vi "Begin.vi"(8 "error in":errorcluster) -> (0 "error out":errorcluster)   [LabVIEW 2018]
doc: "Called before other user functions, this VI is expected to open initial I/O refnums, load in file data, and do all program initialization. Notice that the <B>error out</B> terminal is simply used for data flow. Wiring it to other structures or subVIs ensures that this VI runs first."
uses:
  <vilib>/Rock Robotics/WPI/DriverStation/WPI_DriverStationRobotMode2.ctl
  <vilib>/Rock Robotics/WPI/Joystick/WPI_JoystickDeviceEnum.ctl
  <vilib>/Rock Robotics/WPI/Solenoid/WPI_SolenoidChannel.ctl
  <vilib>/Rock Robotics/SystemInterfaces/DIO/FPGA_DIOChannel.ctl
  <vilib>/Rock Robotics/SystemInterfaces/DIO/FPGA_DIOPWMChannel.ctl
  Robot Global Data.vi
  <vilib>/Rock Robotics/WPI/Solenoid/WPI_SolenoidOpenSingle.vi
  <vilib>/Rock Robotics/WPI/Switch/WPI_SwitchOpenLimit.vi
  <vilib>/Rock Robotics/WPI/Utilities/WPI_GetSetVariantRefNum.vi
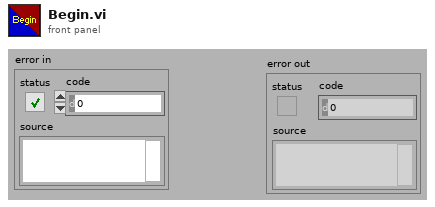
[diagram p1: front panel]
types:
  T1 = typedef "FPGA_DIOPWMChannel.ctl" = enum8{"PWM 0", "PWM 1", "PWM 2", "PWM 3", "PWM 4", "PWM 5", "PWM 6", "PWM 7", "PWM 8", "PWM 9", "PWM MXP 0", "PWM MXP 1", "PWM MXP 2", "PWM MXP 3", "PWM MXP 4", "PWM MXP 5", "PWM MXP 6", "PWM MXP 7", "PWM MXP 8", "PWM MXP 9", "Invalid"}
  T2 = typedef "FPGA_DIOChannel.ctl" = enum8{"DIO 0", "DIO 1", "DIO 2", "DIO 3", "DIO 4", "DIO 5", "DIO 6", "DIO 7", "DIO 8", "DIO 9", "DIO MXP 0", "DIO MXP 1", "DIO MXP 2", "DIO MXP 3", "DIO MXP 4", "DIO MXP 5", "DIO MXP 6", "DIO MXP 7", "DIO MXP 8", "DIO MXP 9", "DIO MXP 10", "DIO MXP 11", "DIO MXP 12", "DIO MXP 13", "DIO MXP 14", "DIO MXP 15", "SPI Port CS1", "SPI Port CS2", "SPI Port CS3", "SPI Port MISO", "SPI Port MOSI", "Invalid"}
  T3 = typedef "WPI_SolenoidChannel.ctl" = enum8{"Solenoid 0", "Solenoid 1", "Solenoid 2", "Solenoid 3", "Solenoid 4", "Solenoid 5", "Solenoid 6", "Solenoid 7", "Invalid"}
  T4 = typedef "WPI_JoystickDeviceEnum.ctl" = enum16{"USB 0", "USB 1", "USB 2", "USB 3", "USB 4", "USB 5"}
  T5 = typedef "WPI_DriverStationRobotMode2.ctl" = enum16{"Autonomous Disabled", "Autonomous Enabled", "Teleop Disabled", "Teleop Enabled", "Disconnected", "Finish", "Test Disabled", "Test Enabled", "Emergency Stopped"}
  T6 = typedef "WPI_MotorControlDeviceRef.ctl" = cluster{"DeviceStatus":errorcluster, "Type":T7, "PWM":cluster{"PWM Channel":T1, "DeadBand":T8}, "CAN":cluster{"Device Number":u8, "SetOutput VI Ref":variant, "GetOutput VI Ref":variant, "Enable VI Ref":variant, "Disable VI Ref":variant, "Data":variant}, "Invert":bool, "DIO PWM":cluster{"PWM \"Enable\" Channel":T1, "DIOChannel":T2, "PWM Rate":dbl}}
  T7 = typedef "WPI_MotorControlType.ctl" = enum16{"PWM", "CAN", "DIO PWM"}
  T8 = typedef "WPI_PWMDeadband.ctl" = cluster{"Name":string, "maxPositivePwm":i32, "minPositivePwm":i32, "centerPwm":i32, "maxNegativePwm":i32, "minNegativePwm":i32, "angularRange":u16}
  T9 = typedef "WPI_JoystickDevRef.ctl" = cluster{"Device":T4}
  T10 = typedef "WPI_SwitchDevRef.ctl" = cluster{"DevStatus":errorcluster, "DIO Channel":T2, "CntIndex":T11, "Normally Closed":bool}
  T11 = typedef "FPGA_CounterCtrSystemIndex.ctl" = enum8{"Ctr 0", "Ctr 1", "Ctr 2", "Ctr 3", "Ctr 4", "Ctr 5", "Ctr 6", "Ctr 7", "Invalid"}
  T12 = typedef "WPI_CompressorDevRef.ctl" = cluster{"DevStatus":errorcluster, "Pneumatics Control Module":u8}
  T13 = typedef "WPI_SolenoidDevRef.ctl" = cluster{"DevStatus":errorcluster, "Pneumatics Control Module":u8, "Forward Solenoid Channel":T3, "Reverse Solenoid Channel":T3}
  T14 = typedef "WPI_PWMDeviceRef.ctl" = cluster{"DeviceStatus":errorcluster, "PWM Channel":T1}
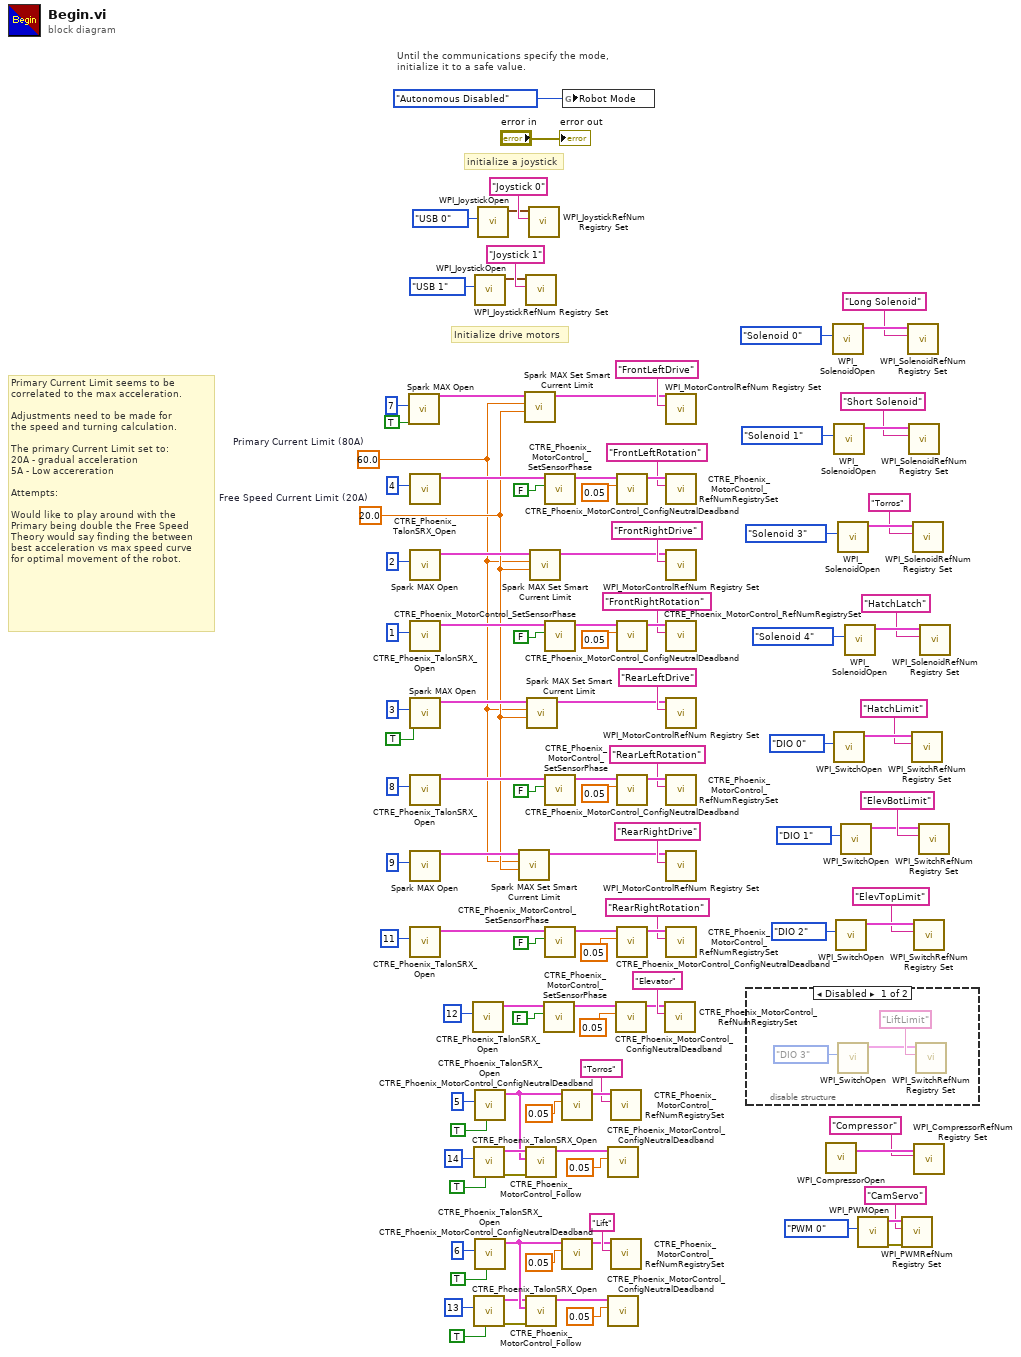
[diagram p0: block diagram]
diagram:
  w1 = 60.0  # Primary Current Limit (80A)
  w2 = 20.0  # Free Speed Current Limit (20A)
  # "Primary Current Limit seems to be\ncorrelated to the max acceleration.\n\nAdjustments need to be made for\nthe speed and turning calculation.\n\nThe primary Current Limit set to:\n20A - gradual acceleration\n5A - Low accereration\n\nAttempts:\n\nWould like to play around with the\nPrimary being double the Free Speed\nTheory would say finding the between\nbest acceleration vs max speed curve\nfor optimal movement of the robot."
  # "Initialize drive motors"
  # "initialize a joystick"
  # "Until the communications specify the mode,\ninitialize it to a safe value."
  n1 = call <vilib>:"Spark MAX Open.vi"("Invert"=TRUE, "Device Number"=u8 7) -> ("MotorControlDeviceRef"=w13:T6)  [unwired: 8 in, 1 out]
  n2 = call <vilib>:"CTRE_Phoenix_TalonSRX_Open.vi"("Device Number"=u8 4) -> ("CAN Talon SRX Ref"=w105:T6)  [unwired: 9 in, 1 out]
  n3 = call <vilib>:"Spark MAX Open.vi"("Device Number"=u8 2) -> ("MotorControlDeviceRef"=w15:T6)  [unwired: 9 in, 1 out]
  n4 = call <vilib>:"CTRE_Phoenix_TalonSRX_Open.vi"("Device Number"=u8 1) -> ("CAN Talon SRX Ref"=w98:T6)  [unwired: 9 in, 1 out]
  n5 = call <vilib>:"Spark MAX Open.vi"("Invert"=TRUE, "Device Number"=u8 3) -> ("MotorControlDeviceRef"=w11:T6)  [unwired: 8 in, 1 out]
  n6 = call <vilib>:"CTRE_Phoenix_TalonSRX_Open.vi"("Device Number"=u8 8) -> ("CAN Talon SRX Ref"=w91:T6)  [unwired: 9 in, 1 out]
  n7 = call <vilib>:"Spark MAX Open.vi"("Device Number"=u8 9) -> ("MotorControlDeviceRef"=w9:T6)  [unwired: 9 in, 1 out]
  n8 = call <vilib>:"CTRE_Phoenix_TalonSRX_Open.vi"("Device Number"=u8 11) -> ("CAN Talon SRX Ref"=w78:T6)  [unwired: 9 in, 1 out]
  n9 = call <vilib>:"CTRE_Phoenix_TalonSRX_Open.vi"("Device Number"=u8 12) -> ("CAN Talon SRX Ref"=w60:T6)  [unwired: 9 in, 1 out]
  n10 = call <vilib>:"CTRE_Phoenix_TalonSRX_Open.vi"("Invert"=TRUE, "Device Number"=u8 14) -> ("error out"=w43:errorcluster, "CAN Talon SRX Ref"=w42:T6)  [unwired: 8 in]
  n11 = call <vilib>:"CTRE_Phoenix_TalonSRX_Open.vi"("Invert"=TRUE, "Device Number"=u8 13) -> ("error out"=w28:errorcluster, "CAN Talon SRX Ref"=w29:T6)  [unwired: 8 in]
  n12 = call <vilib>:"WPI_JoystickOpen.vi"("JoystickDevice"=WPI_JoystickDeviceEnum."USB 1") -> ("JoystickDevRef"=w75:T9)  [unwired: 10 in]
  n13 = call <vilib>:"CTRE_Phoenix_TalonSRX_Open.vi"("Invert"=TRUE, "Device Number"=u8 5) -> ("CAN Talon SRX Ref"=w41:T6)  [unwired: 8 in, 1 out]
  n14 = call <vilib>:"CTRE_Phoenix_TalonSRX_Open.vi"("Invert"=TRUE, "Device Number"=u8 6) -> ("CAN Talon SRX Ref"=w30:T6)  [unwired: 8 in, 1 out]
  n15 = call <vilib>:"WPI_JoystickOpen.vi"("JoystickDevice"=WPI_JoystickDeviceEnum."USB 0") -> ("JoystickDevRef"=w112:T9)  [unwired: 10 in]
  n16 = call <vilib>:"Spark MAX Set Smart Current Limit.vi"("Free Speed Current Limit (20A)"=w2, "Primay Current Limit (80A)"=w1, "MotorControlDeviceRef in"=w9) -> ("MotorControlDeviceRef out"=w8:T6)  [unwired: 7 in, 1 out]
  n17 = call <vilib>:"Spark MAX Set Smart Current Limit.vi"("Free Speed Current Limit (20A)"=w2, "Primay Current Limit (80A)"=w1, "MotorControlDeviceRef in"=w13) -> ("MotorControlDeviceRef out"=w12:T6)  [unwired: 7 in, 1 out]
  n18 = call <vilib>:"WPI_JoystickRefNum Registry Set.vi"("refnum name"="Joystick 1", "JoystickDevRef"=w75) -> ()  [unwired: 8 in, 2 out]
  n19 = call <vilib>:"CTRE_Phoenix_MotorControl_Follow.vi"("error in (no error)"=w43, "Master Controller to Follow"=w41, "PhoenixMotorControlDevRef"=w42) -> ("PhoenixMotorControlDevRef"=w40:T6)  [unwired: 7 in, 1 out]
  n20 = call <vilib>:"CTRE_Phoenix_MotorControl_Follow.vi"("error in (no error)"=w28, "Master Controller to Follow"=w30, "PhoenixMotorControlDevRef"=w29) -> ("PhoenixMotorControlDevRef"=w31:T6)  [unwired: 7 in, 1 out]
  n21 = call <vilib>:"Spark MAX Set Smart Current Limit.vi"("Free Speed Current Limit (20A)"=w2, "Primay Current Limit (80A)"=w1, "MotorControlDeviceRef in"=w11) -> ("MotorControlDeviceRef out"=w10:T6)  [unwired: 7 in, 1 out]
  n22 = call <vilib>:"WPI_JoystickRefNum Registry Set.vi"("refnum name"="Joystick 0", "JoystickDevRef"=w112) -> ()  [unwired: 8 in, 2 out]
  n23 = call <vilib>:"Spark MAX Set Smart Current Limit.vi"("Free Speed Current Limit (20A)"=w2, "Primay Current Limit (80A)"=w1, "MotorControlDeviceRef in"=w15) -> ("MotorControlDeviceRef out"=w14:T6)  [unwired: 7 in, 1 out]
  n24 = call <vilib>:"CTRE_Phoenix_MotorControl_SetSensorPhase.vi"("PhaseSensor"=FALSE, "PhoenixMotorControlDevRef"=w60) -> ("PhoenixMotorControlDevRef"=w57:T6)  [unwired: 8 in, 1 out]
  n25 = call <vilib>:"CTRE_Phoenix_MotorControl_SetSensorPhase.vi"("PhaseSensor"=FALSE, "PhoenixMotorControlDevRef"=w105) -> ("PhoenixMotorControlDevRef"=w106:T6)  [unwired: 8 in, 1 out]
  n26 = call <vilib>:"CTRE_Phoenix_MotorControl_SetSensorPhase.vi"("PhaseSensor"=FALSE, "PhoenixMotorControlDevRef"=w98) -> ("PhoenixMotorControlDevRef"=w97:T6)  [unwired: 8 in, 1 out]
  n27 = call <vilib>:"CTRE_Phoenix_MotorControl_SetSensorPhase.vi"("PhaseSensor"=FALSE, "PhoenixMotorControlDevRef"=w91) -> ("PhoenixMotorControlDevRef"=w92:T6)  [unwired: 8 in, 1 out]
  n28 = call <vilib>:"CTRE_Phoenix_MotorControl_SetSensorPhase.vi"("PhaseSensor"=FALSE, "PhoenixMotorControlDevRef"=w78) -> ("PhoenixMotorControlDevRef"=w86:T6)  [unwired: 8 in, 1 out]
  n29 = call <vilib>:"CTRE_Phoenix_MotorControl_ConfigNeutralDeadband.vi"("Percent Deadband"=0.05, "PhoenixMotorControlDevRef"=w41) -> ("PhoenixMotorControlDevRef"=w48:T6)  [unwired: 8 in, 1 out]
  n30 = call <vilib>:"CTRE_Phoenix_MotorControl_ConfigNeutralDeadband.vi"("Percent Deadband"=0.05, "PhoenixMotorControlDevRef"=w30) -> ("PhoenixMotorControlDevRef"=w23:T6)  [unwired: 8 in, 1 out]
  n31 = global write "Robot Global Data.vi" "Robot Mode"(WPI_DriverStationRobotMode2."Autonomous Disabled" ("Robot Mode")) -> ()
  n32 = call <vilib>:"CTRE_Phoenix_MotorControl_ConfigNeutralDeadband.vi"("Percent Deadband"=0.05, "PhoenixMotorControlDevRef"=w40) -> ()  [unwired: 8 in, 2 out]
  n33 = call <vilib>:"CTRE_Phoenix_MotorControl_ConfigNeutralDeadband.vi"("Percent Deadband"=0.05, "PhoenixMotorControlDevRef"=w31) -> ()  [unwired: 8 in, 2 out]
  n34 = call <vilib>:"CTRE_Phoenix_MotorControl_RefNumRegistrySet.vi"("refnum name"="Torros", "PhoenixMotorControlDevRef"=w48) -> ()  [unwired: 8 in, 2 out]
  n35 = call <vilib>:"CTRE_Phoenix_MotorControl_RefNumRegistrySet.vi"("refnum name"="Lift", "PhoenixMotorControlDevRef"=w23) -> ()  [unwired: 8 in, 2 out]
  n36 = call <vilib>:"CTRE_Phoenix_MotorControl_ConfigNeutralDeadband.vi"("Percent Deadband"=0.05, "PhoenixMotorControlDevRef"=w57) -> ("PhoenixMotorControlDevRef"=w58:T6)  [unwired: 8 in, 1 out]
  n37 = call <vilib>:"CTRE_Phoenix_MotorControl_ConfigNeutralDeadband.vi"("Percent Deadband"=0.05, "PhoenixMotorControlDevRef"=w106) -> ("PhoenixMotorControlDevRef"=w104:T6)  [unwired: 8 in, 1 out]
  n38 = call <vilib>:"CTRE_Phoenix_MotorControl_ConfigNeutralDeadband.vi"("Percent Deadband"=0.05, "PhoenixMotorControlDevRef"=w97) -> ("PhoenixMotorControlDevRef"=w99:T6)  [unwired: 8 in, 1 out]
  n39 = call <vilib>:"CTRE_Phoenix_MotorControl_ConfigNeutralDeadband.vi"("Percent Deadband"=0.05, "PhoenixMotorControlDevRef"=w92) -> ("PhoenixMotorControlDevRef"=w90:T6)  [unwired: 8 in, 1 out]
  n40 = call <vilib>:"CTRE_Phoenix_MotorControl_ConfigNeutralDeadband.vi"("Percent Deadband"=0.05, "PhoenixMotorControlDevRef"=w86) -> ("PhoenixMotorControlDevRef"=w85:T6)  [unwired: 8 in, 1 out]
  n41 = call <vilib>:"CTRE_Phoenix_MotorControl_RefNumRegistrySet.vi"("refnum name"="Elevator", "PhoenixMotorControlDevRef"=w58) -> ()  [unwired: 8 in, 2 out]
  n42 = call <vilib>:"WPI_MotorControlRefNum Registry Set.vi"("refnum name"="FrontLeftDrive", "MotorControlDevRef"=w12) -> ()  [unwired: 8 in, 2 out]
  n43 = call <vilib>:"CTRE_Phoenix_MotorControl_RefNumRegistrySet.vi"("refnum name"="FrontLeftRotation", "PhoenixMotorControlDevRef"=w104) -> ()  [unwired: 8 in, 2 out]
  n44 = call <vilib>:"WPI_MotorControlRefNum Registry Set.vi"("refnum name"="FrontRightDrive", "MotorControlDevRef"=w14) -> ()  [unwired: 8 in, 2 out]
  n45 = call <vilib>:"CTRE_Phoenix_MotorControl_RefNumRegistrySet.vi"("refnum name"="FrontRightRotation", "PhoenixMotorControlDevRef"=w99) -> ()  [unwired: 8 in, 2 out]
  n46 = call <vilib>:"WPI_MotorControlRefNum Registry Set.vi"("refnum name"="RearLeftDrive", "MotorControlDevRef"=w10) -> ()  [unwired: 8 in, 2 out]
  n47 = call <vilib>:"CTRE_Phoenix_MotorControl_RefNumRegistrySet.vi"("refnum name"="RearLeftRotation", "PhoenixMotorControlDevRef"=w90) -> ()  [unwired: 8 in, 2 out]
  n48 = call <vilib>:"WPI_MotorControlRefNum Registry Set.vi"("refnum name"="RearRightDrive", "MotorControlDevRef"=w8) -> ()  [unwired: 8 in, 2 out]
  n49 = call <vilib>:"CTRE_Phoenix_MotorControl_RefNumRegistrySet.vi"("refnum name"="RearRightRotation", "PhoenixMotorControlDevRef"=w85) -> ()  [unwired: 8 in, 2 out]
  n50 = disable-structure shown="Disabled" {
    frame Disabled {
      n51 = call-poly <vilib>:"WPI_SwitchOpen.vi"("DIO Channel"=FPGA_DIOChannel."DIO 3") -> ("SwitchDevRef"=w115:T10)  [unwired: 9 in, 1 out]
      n52 = call <vilib>:"WPI_SwitchRefNum Registry Set.vi"("refnum name"="LiftLimit", "SwitchDevRef"=w115) -> ()  [unwired: 8 in, 2 out]
    }
    frame Enabled {
    }
  }
  n53 = call <vilib>:"WPI_CompressorOpen.vi"() -> ("CompressorDevRef"=w51:T12)  [unwired: 14 in, 1 out]
  n54 = call-poly <vilib>:"WPI_SolenoidOpen.vi"("Solenoid Channel"=WPI_SolenoidChannel."Solenoid 0") -> ("SolenoidDevRef"=w71:T13)  [unwired: 9 in, 1 out]
  n55 = call-poly <vilib>:"WPI_SolenoidOpen.vi"("Solenoid Channel"=WPI_SolenoidChannel."Solenoid 1") -> ("SolenoidDevRef"=w72:T13)  [unwired: 9 in, 1 out]
  n56 = call-poly <vilib>:"WPI_SwitchOpen.vi"("DIO Channel"=FPGA_DIOChannel."DIO 0") -> ("SwitchDevRef"=w54:T10)  [unwired: 9 in, 1 out]
  n57 = call-poly <vilib>:"WPI_SwitchOpen.vi"("DIO Channel"=FPGA_DIOChannel."DIO 2") -> ("SwitchDevRef"=w36:T10)  [unwired: 9 in, 1 out]
  n58 = call-poly <vilib>:"WPI_SolenoidOpen.vi"("Solenoid Channel"=WPI_SolenoidChannel."Solenoid 3") -> ("SolenoidDevRef"=w65:T13)  [unwired: 9 in, 1 out]
  n59 = call-poly <vilib>:"WPI_SwitchOpen.vi"("DIO Channel"=FPGA_DIOChannel."DIO 1") -> ("SwitchDevRef"=w37:T10)  [unwired: 9 in, 1 out]
  n60 = call-poly <vilib>:"WPI_SolenoidOpen.vi"("Solenoid Channel"=WPI_SolenoidChannel."Solenoid 4") -> ("SolenoidDevRef"=w67:T13)  [unwired: 9 in, 1 out]
  n61 = call <vilib>:"WPI_PWMOpen.vi"("PWM Channel"=FPGA_DIOPWMChannel."PWM 0") -> ("error out"=w21:errorcluster, "PWMDeviceRef"=w20:T14)  [unwired: 9 in]
  n62 = call <vilib>:"WPI_PWMRefNum Registry Set.vi"("error in (no error)"=w21, "refnum name"="CamServo", "PWMDeviceRef"=w20) -> ()  [unwired: 7 in, 2 out]
  n63 = call <vilib>:"WPI_SolenoidRefNum Registry Set.vi"("refnum name"="Long Solenoid", "SolenoidDevRef"=w71) -> ()  [unwired: 8 in, 2 out]
  n64 = call <vilib>:"WPI_SolenoidRefNum Registry Set.vi"("refnum name"="Short Solenoid", "SolenoidDevRef"=w72) -> ()  [unwired: 8 in, 2 out]
  n65 = call <vilib>:"WPI_SwitchRefNum Registry Set.vi"("refnum name"="HatchLimit", "SwitchDevRef"=w54) -> ()  [unwired: 8 in, 2 out]
  n66 = call <vilib>:"WPI_SolenoidRefNum Registry Set.vi"("refnum name"="Torros", "SolenoidDevRef"=w65) -> ()  [unwired: 8 in, 2 out]
  n67 = call <vilib>:"WPI_SwitchRefNum Registry Set.vi"("refnum name"="ElevTopLimit", "SwitchDevRef"=w36) -> ()  [unwired: 8 in, 2 out]
  n68 = call <vilib>:"WPI_CompressorRefNum Registry Set.vi"("refnum name"="Compressor", "CompressorDevRef"=w51) -> ()  [unwired: 8 in, 2 out]
  n69 = call <vilib>:"WPI_SwitchRefNum Registry Set.vi"("refnum name"="ElevBotLimit", "SwitchDevRef"=w37) -> ()  [unwired: 8 in, 2 out]
  n70 = call <vilib>:"WPI_SolenoidRefNum Registry Set.vi"("refnum name"="HatchLatch", "SolenoidDevRef"=w67) -> ()  [unwired: 8 in, 2 out]
  "error out" <- "error in"
